vi "Update Log File Progress.vi"(8 "Bytes Downloaded":i32, 9 "File Size":i32, 10 "Selected index":i32, 11 "Log files":T1[](array[typedef])) -> (3 "Log File Out":T1[](array[typedef]))   [LabVIEW 2019]
uses:
  Controls/Log State.ctl
  Controls/Log.ctl
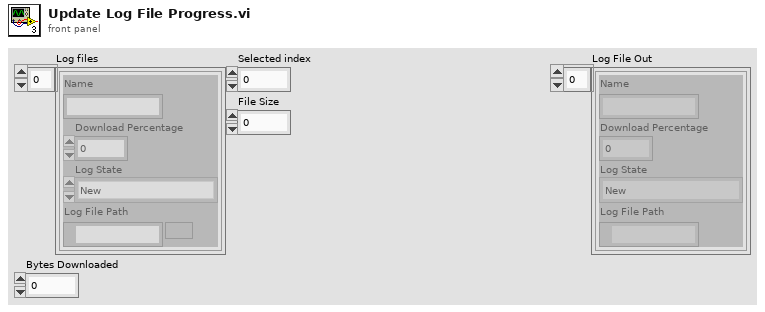
[diagram p1: front panel]
types:
  T1 = typedef "Log.ctl" = cluster{"Name":string, "Download Percentage":dbl, "Log State":T2, "Log File Path":path}
  T2 = typedef "Log State.ctl" = enum16{"New", "Downloading", "Downloaded"}
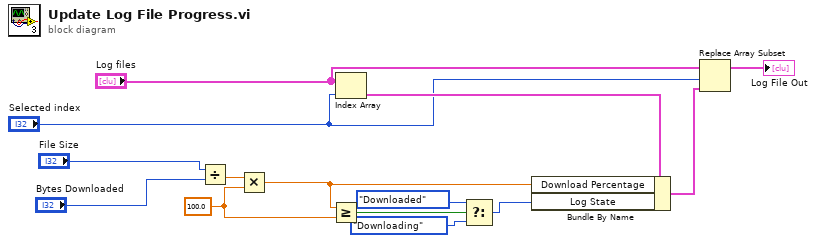
[diagram p0: block diagram]
diagram:
  w5 = 100.0 ("y")
  n1 = Divide(x="File Size", y="Bytes Downloaded") -> (x/y=w11:dbl)
  n2 = Multiply(x=w11, y=w5) -> (x*y=w6:dbl)
  n3 = Greater Or Equal?(x=w6, y=w5) -> (x >= y?=w4:bool)
  n4 = Index Array(array="Log files", index="Selected index") -> (element=w14:T1)
  n5 = Select(t=Log_State."Downloaded" ("Log State"), s=w4, f=Log_State."Downloading" ("Log State")) -> (s? t:f=w1:T2)
  n6 = Bundle By Name(cluster=w14, "Download Percentage"=w6, "Log State"=w1) -> (w9:T1)
  n7 = Replace Array Subset(array="Log files", new element=w9, index="Selected index") -> (→"Log File Out":T1[])
